vi "EditOptions.vi"(8 "error in":errorcluster, 11 "node in":refnum<class "Targets.lvclass">) -> (0 "error out":errorcluster, 1 "edit options":T1, 2 "subnodes class":T2, 3 "node out":refnum<class "Targets.lvclass">)   [LabVIEW 2015, in "Targets.lvclass"]
doc: "Contains the options for the Menu that will be displayed when doing right click on an item.\nThe sub nodes class configures which nodes can be added to this nodes\nAnd the edit options determine which options are available for the node.\nThis configuration is stored in this VI in case some dynamic configuration is required for the menu options or sub nodes."
uses:
  Targets.lvclass
  <vilib>/NI/Configuration Framework/Node/SubNodeCluster.ctl
  <vilib>/NI/Configuration Framework/Node/NodeMenuOptions.ctl
  <vilib>/NI/Configuration Framework/Node/NISE_CEF_Node.lvclass/NISE_CEF_Node.ctl
  Target/Target.lvclass
  Target/Target.lvclass/Target.ctl
  Target/Read Source.vi
  <vilib>/NI/Configuration Framework/Node/ReadChildren.vi
  <vilib>/NI/Configuration Framework/Node/NISE_CEF_Node.lvclass
  Configuration Tool.lvlib
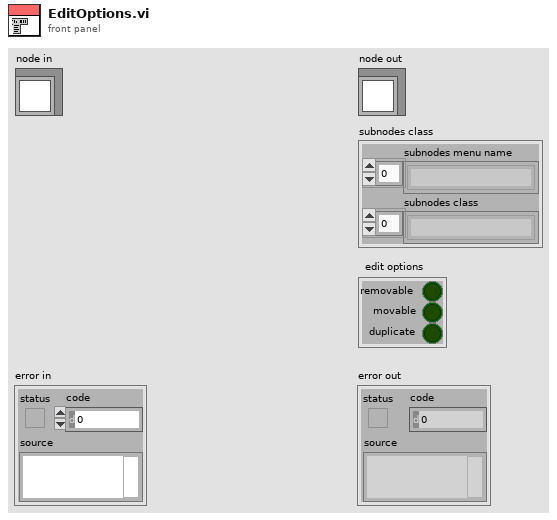
[diagram p1: front panel]
types:
  T1 = typedef "NISE_CEF_Node.lvclass/NodeMenuOptions.ctl" = cluster{"removable":bool, "movable":bool, "duplicate":bool}
  T2 = typedef "NISE_CEF_Node.lvclass/SubNodeCluster.ctl" = cluster{"subnodes menu name":string[], "subnodes class":string[]}
  T3 = typedef "NISE_CEF_Node.lvclass/NodeRef.ctl" = refnum<data-value>
  T4 = typedef "Configuration Tool.lvlib/Path Cluster.ctl" = cluster{"Path":path, "Path Type":enum16{"Absolute", "To Base", "To Common Doc Dir", "To Application Data Dir"}}
  T5 = typedef "Configuration Tool.lvlib/Target.ctl" = enum16{"All", "Pharlap", "VxWorks", "Windows", "Linux_32_ARM", "Linux_x64", "PharlapWindows", "PharlapVxWorks", "VxWorksWindows"}
  T6 = cluster{"Source":T4, "Real Time System Destination":string, "Supported Target":T5}
  T7 = enum16{"All", "Pharlap", "VxWorks", "Windows", "Linux_32_ARM", "Linux_x64", "PharlapWindows", "PharlapVxWorks", "VxWorksWindows"}[]
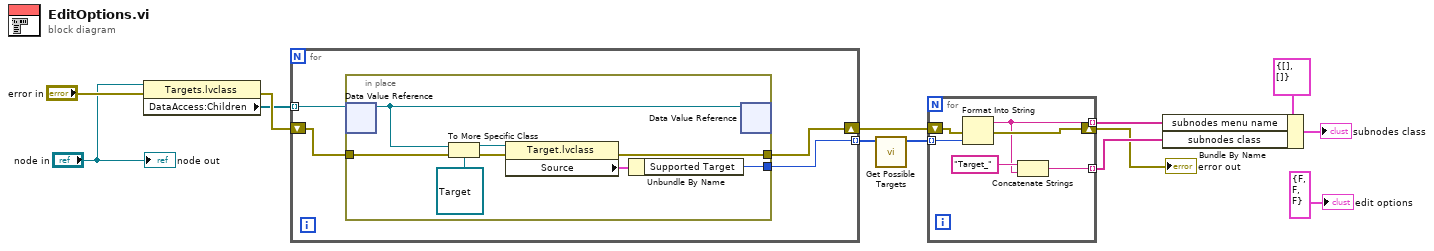
[diagram p0: block diagram]
diagram:
  n1 = property class="Targets.lvclass"(reference="node in", error in="error in") -> (error out=w9:errorcluster, "DataAccess:Children"=w8:T3[])  [unwired: 1 out]
  n2 = for {
    shift-right: [w14] -> w6
    shift-left: w9 -> [w15]
    tunnel: w8 -> [w17] mode=indexing
    tunnel: [w16] -> w7 mode=indexing
    n3 = in-place {
      in-place-border: [w21] -> w16
      in-place-border: w15 -> [w20]
      in-place-border: [w18] -> w14
      n4 = in-place-dvr #1(w17) -> (w24:refnum<class "NISE_CEF_Node.lvclass">)  [unwired: 1 out]
      n5 = To More Specific Class(target class=refnum<class "Target.lvclass"> refnum ("Target.lvclass"), reference=w24, error in=w20) -> (specific class reference=w22:refnum<class "Target.lvclass">, error out=w19:errorcluster)
      n6 = property class="Target.lvclass"(reference=w22, error in=w19) -> (error out=w18:errorcluster, "Source"=w23:T6)  [unwired: 1 out]
      n7 = Unbundle By Name(w23) -> ("Supported Target"=w21:T5)
      n8 = in-place-dvr #1(w24) -> ()  [unwired: 2 out]
    }
  }
  n9 = call "Get Possible Targets.vi"("Targets Used"=w7) -> ("Possible Targets"=w5:T7)  [unwired: 10 in]
  n10 = for {
    shift-right: [w29] -> w1
    shift-left: w6 -> [w30]
    tunnel: w5 -> [w31] mode=indexing
    tunnel: [w27] -> w4 mode=indexing
    tunnel: [w26] -> w2 mode=indexing
    n11 = Format Into String(error in=w30, w31) -> (resulting string=w27:string, error out=w29:errorcluster)  [unwired: 2 in]
    n12 = Concatenate Strings("Target_" ("Class"), w27) -> (w26:string)
  }
  "error out" <- w1
  n13 = Bundle By Name(cluster=T2 {"subnodes menu name"=[], "subnodes class"=[]} ("subnodes class"), "subnodes menu name"=w4, "subnodes class"=w2) -> (→"subnodes class":T2)
  "node out" <- "node in"
  "edit options" <- T1 {"removable"=FALSE, "movable"=FALSE, "duplicate"=FALSE} ("edit options")
